vi "TxAM.vi"() -> ()   [LabVIEW 2012]
uses:
  <vilib>/measure/NI_MAPro.lvlib
  <instrlib>/niUSRP/niUSRP Write Tx Data (CDB).vi
  <vilib>/Analysis/NI_AALBase.lvlib
  <vilib>/Analysis/baseanly.llb/Quick Scale 1D.vi
panel:
  out "Baseband Signal":dbl[](graph)
  out "Message":waveform(dbl)(graph)
  out "error out":errorcluster
  in  "stop":bool
  in  "Modulation index":dbl=1.0 min=0.0 max=1.0
  in  "#tones":i32=3
  in  "delta frequency":dbl=1000.0 format="%.2p"
  in  "start frequency":dbl=1000.0 format="%.2p"
  in  "message length (samples)":dbl=200000.0
  in  "active antenna":string="TX1"
  out "actual gain (dB)":dbl format="%#_6f"
  in  "gain (dB)":dbl format="%#_6f"
  out "actual carrier frequency":dbl=100000.0 format="%#_6p"
  in  "carrier frequency":dbl=915100000.0 format="%#_6p"
  out "actual IQ rate":dbl=100000.0 format="%#_6p"
  in  "IQ rate":dbl=200000.0 format="%#_6p"
  in  "device names":refnum<k15>="192.168.10.2"
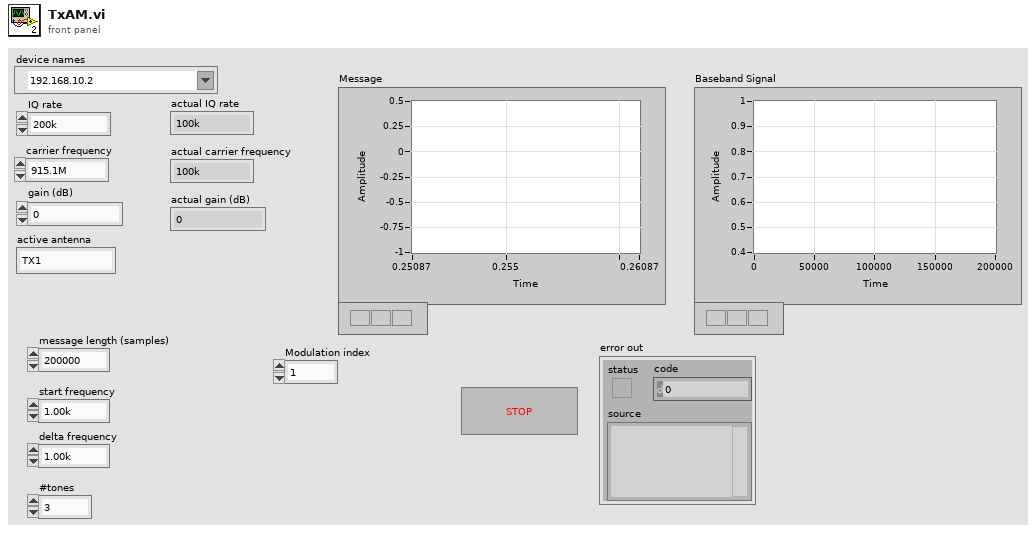
[diagram p1: front panel]
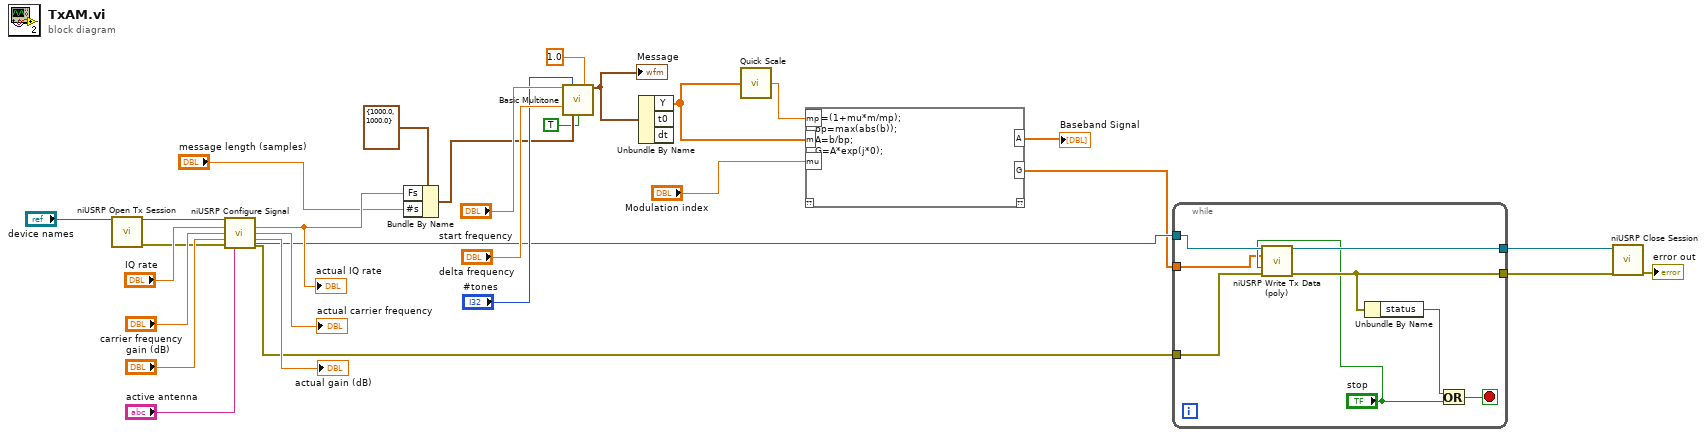
[diagram p0: block diagram]
diagram:
  n1 = call <instrlib>:"niUSRP Open Tx Session.vi"("device names"="device names") -> ("session handle out"=w28:refnum<k15>, "error out"=w22:errorcluster)  [unwired: 13 in]
  n2 = call <instrlib>:"niUSRP Configure Signal.vi"("session handle"=w28, "IQ rate"="IQ rate", "carrier frequency"="carrier frequency", "gain"="gain (dB)", "error in (no error)"=w22, "active antenna"="active antenna") -> ("session handle out"=w12:refnum<k15>, "coerced IQ rate"=w19:dbl, "coerced carrier frequency"=→"actual carrier frequency":dbl, "coerced gain"=→"actual gain (dB)":dbl, "error out"=w10:errorcluster)  [unwired: 5 in]
  "actual IQ rate" <- w19
  n3 = Bundle By Name(cluster=cluster{"Fs":dbl, "#s":dbl} {"Fs"=1000.0, "#s"=1000.0} ("sampling info"), "Fs"=w19, "#s"="message length (samples)") -> (w13:cluster{"Fs":dbl, "#s":dbl})
  n4 = call <vilib>:"Basic Multitone.vi"("start frequency"="start frequency", "#tones"="#tones", "amplitude"=1.0, "delta frequency"="delta frequency", "sampling info"=w13, "coerce frequencies?"=TRUE) -> ("signal out"=w3:waveform(dbl))  [unwired: 6 in, 3 out]
  "Message" <- w3
  n5 = Unbundle By Name(w3) -> ("Y"=w5:dbl[])  [unwired: 2 out]
  n6 = call-poly <vilib>:"Quick Scale.vi"("X"=w5) -> ("max|X|"=w4:dbl)  [unwired: 2 out]
  n7 = mathscript code="b=(1+mu*m/mp);\nbp=max(abs(b));\nA=b/bp;\nG=A*exp(j*0);"("mp"=w4, "m"=w5, "mu"="Modulation index") -> ("A"=→"Baseband Signal":dbl[], "G"=w6:cdb[])  [unwired: 1 in, 1 out]
  n8 = while {
    tunnel: w12 -> [w37]
    tunnel: [w36] -> w11
    tunnel: w10 -> [w35]
    tunnel: [w34] -> w9
    tunnel: w6 -> [w30]
    stop <- w32 stop-if-true
    n9 = call-poly <instrlib>:"niUSRP Write Tx Data (poly).vi"("session handle"=w37, "data"=w30, "end of data?"="stop", "error in (no error)"=w35) -> ("session handle out"=w36:refnum<k15>, "error out"=w34:errorcluster)  [unwired: 10 in]
    n10 = Unbundle By Name(w34) -> ("status"=w33:bool)
    n11 = Or(x=w33, y="stop") -> (x .or. y?=w32:bool)
  }
  n12 = call <instrlib>:"niUSRP Close Session.vi"("session handle"=w11, "error in (no error)"=w9) -> ("error out"=→"error out":errorcluster)  [unwired: 13 in]
